vi "poll_lidar.vi"() -> ()   [LabVIEW 2017]
panel:
  out "XY Graph":cluster{dbl[], dbl[]}[](graph)
  out "Distance from Wall":dbl
  in  "stop":bool
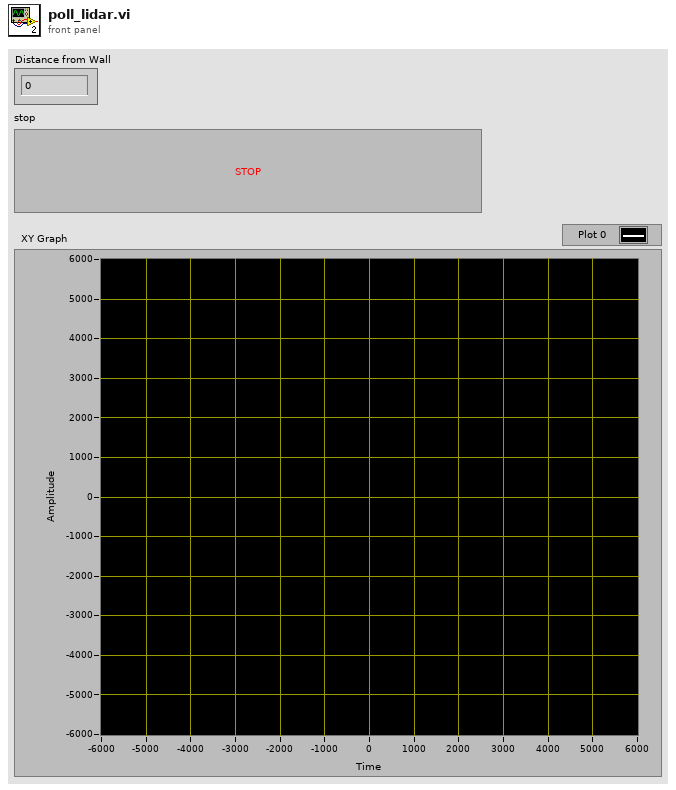
[diagram p1: front panel]
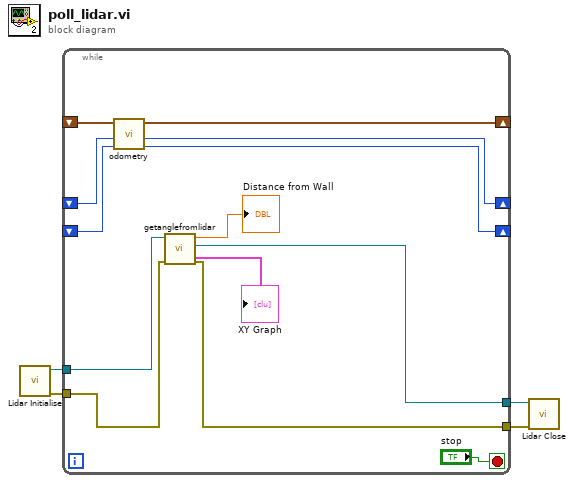
[diagram p0: block diagram]
diagram:
  n1 = call "Lidar Initialise.vi"() -> ("error out"=w4:errorcluster, "VISA resource name out"=w2:refnum<visa-resource-name>)  [unwired: 10 in]
  n2 = while {
    shift-right: [w16] -> _
    shift-left: _ -> [w14]
    shift-right: [w15] -> _
    shift-left: _ -> [w13]
    shift-right: [w12] -> _
    shift-left: _ -> [w11]
    tunnel: w4 -> [w9]
    tunnel: [w8] -> w3
    tunnel: w2 -> [w10]
    tunnel: [w7] -> w1
    stop <- "stop" stop-if-true
    n3 = call "odometry.vi"("ENCB in"=w13, "ENCA in"=w14, "Position"=w11) -> ("ENCB OUT"=w15:i32, "ENCA OUT"=w16:i32, "X, Y, BEARING"=w12:cluster{dbl, dbl, dbl})  [unwired: 5 in]
    n4 = call "getanglefromlidar.vi"("error in (no error)"=w9, "VISA resource name"=w10) -> ("error constant"=w8:errorcluster, "VISA resource name out"=w7:refnum<visa-resource-name>, "Distance from Wall"=→"Distance from Wall":dbl, "XY Graph"=→"XY Graph":cluster{dbl[], dbl[]}[])  [unwired: 6 in]
  }
  n5 = call "Lidar Close.vi"("error in (no error)"=w3, "VISA resource name"=w1) -> ()  [unwired: 9 in, 1 out]
